vi "GetBooksToGrade.vi"(3 "Value":i32[](array[numeric]), 4 "dropBox":string, 5 "ItemNames":string[][](array[string]), 6 "Paths":T2) -> ()   [LabVIEW 2012]
uses:
  <vilib>/RoboBookEngine/Server/HTTPServer/PathsGlobal.ctl
  <userlib>/BotSpeak/Devices/EvalRIO/FTPCodes/FTPParameters.ctl
panel:
  in  "Parameters":T1={"Book Folder Name"="", "Full file name"="", "Remote Path"="bookfiles/", "Shelf folder"=path "", "Existing books"=[], "Dialog?"=enum."No Dialog", "New Format?"=FALSE}
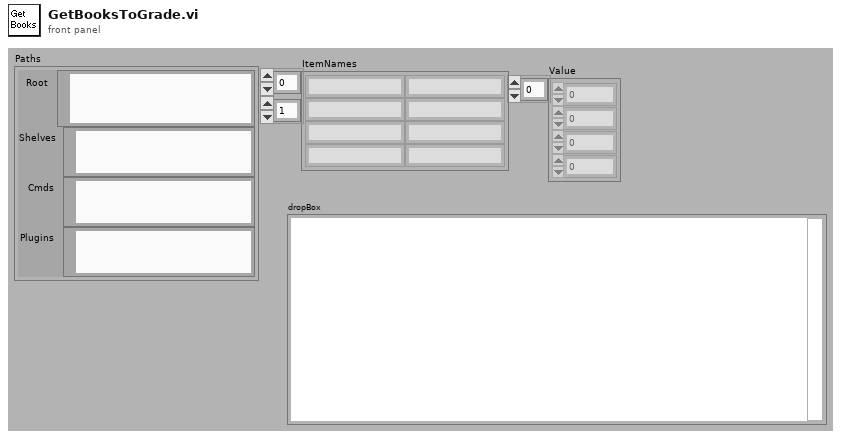
[diagram p1: front panel]
types:
  T1 = typedef "FTPParameters.ctl" = cluster{"Book Folder Name":string, "Full file name":string, "Remote Path":string, "Shelf folder":path, "Existing books":string[], "Dialog?":enum16{"No Dialog", "Dialog", "Overwrite"}, "New Format?":bool}
  T2 = typedef "PathsGlobal.ctl" = cluster{"Root":path, "Shelves":path, "Cmds":path, "Plugins":path}
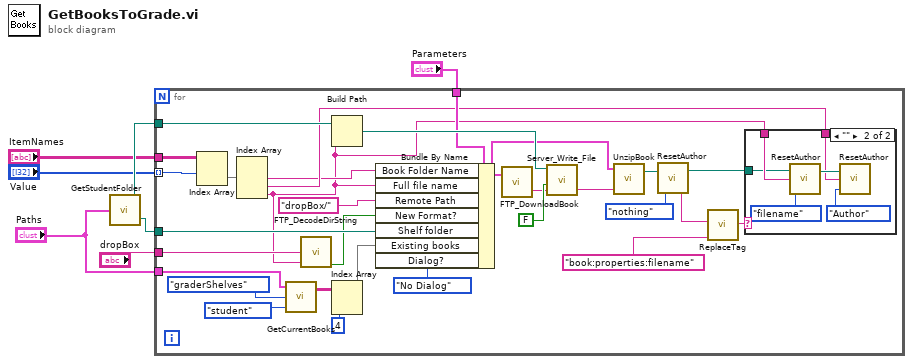
[diagram p0: block diagram]
diagram:
  n1 = call <vilib>:"GetStudentFolder.vi"("Paths"="Paths") -> ("Student"=w7:path, "Graded"=w3:path)
  n2 = for {
    tunnel: "ItemNames" -> [w36]
    tunnel: "Value" -> [w35] mode=indexing
    tunnel: w7 -> [w31]
    tunnel: "Parameters" -> [w29]
    tunnel: w3 -> [w27]
    tunnel: "Paths" -> [w21]
    tunnel: "dropBox" -> [w10]
    n3 = Index Array(array=w36, index (row)=w35) -> (element=w34:string[])  [unwired: 1 in]
    n4 = Index Array(array=w34) -> (element #1=w11:string, element #2=w13:string, element #3=w9:string)  [unwired: 3 in]
    n5 = call <vilib>:"GetCurrentBooks.vi"("user"=enum16{"student", "creator"}."student", "Folder"=enum16{"MyShelves", "graderShelves"}."graderShelves", "Paths"=w21) -> ("books"=w24:string[][])  [unwired: 1 out]
    n6 = call <userlib>:"FTP_DecodeDirString.vi"("directory"=w10, "name"=w9) -> ("New Format?"=w8:bool)  [unwired: 5 out]
    n7 = Build Path(base path=w31, name or relative path=w9) -> (appended path=w30:path)
    n8 = Index Array(array=w24, index (col)=4 ("disabled index (col)")) -> (element=w20:string[])  [unwired: 1 in]
    n9 = Bundle By Name(cluster=w29, "Book Folder Name"=w11, "Full file name"=w9, "Remote Path"="dropBox/", "New Format?"=w8, "Shelf folder"=w27, "Existing books"=w20, "Dialog?"=enum16{"No Dialog", "Dialog", "Overwrite"}."No Dialog") -> (w26:T1)
    n10 = call <userlib>:"FTP_DownloadBook.vi"("Parameters"=w26) -> ("ZipFile"=w28:string)  [unwired: 1 in, 1 out]
    n11 = call <vilib>:"Server_Write_File.vi"("advisory dialog? (display:T)"=FALSE, "character string"=w28, "file path (dialog if empty)"=w30) -> ()  [unwired: 1 in, 3 out]
    n12 = call <vilib>:"UnzipBook.vi"("FileZipped"=w28, "Parameters"=w26) -> ("Book"=w14:path)  [unwired: 1 in, 1 out]
    n13 = call <vilib>:"ResetAuthor.vi"("Update"=enum16{"Author", "filename", "title", "nothing"}."nothing", "BookFolder"=w14) -> ("contents"=w17:string, "BookFolder out"=w15:path)  [unwired: 1 in]
    n14 = call <vilib>:"ReplaceTag.vi"("tag"="book:properties:filename", "contents"=w17) -> ("old tag"=w16:string)  [unwired: 2 in, 1 out]
    n15 = case shown="\"\"" w16 {
      tunnel: w9 -> [_ w41]
      tunnel: w13 -> [_ w38]
      tunnel: w15 -> [_ w37]
      frame Default {
      }
      frame "" {
        n16 = call <vilib>:"ResetAuthor.vi"("Update"=enum16{"Author", "filename", "title", "nothing"}."filename", "new tag"=w41, "BookFolder"=w37) -> ("BookFolder out"=w40:path)  [unwired: 1 out]
        n17 = call <vilib>:"ResetAuthor.vi"("Update"=enum16{"Author", "filename", "title", "nothing"}."Author", "new tag"=w38, "BookFolder"=w40) -> ()  [unwired: 2 out]
      }
    }
  }
